vi "Get Logger Status.vi"(8 "Error In":errorcluster, 9 "Timeout (s)":dbl=10.0 format="%#_13g", 10 "Synchronize with Logger (False)":bool, 11 "TDMS Log In":refnum<class "TDMS Logger.lvclass">) -> (0 "Error Out":errorcluster, 1 "timed out?":bool, 2 "Logger Status":T1, 3 "TDMS Log Out":refnum<class "TDMS Logger.lvclass">)   [LabVIEW 2015, in "TDMS Logger.lvlib" / "TDMS Logger.lvclass"]
doc: "This VI returns the cluster with the status of the data logger. The status contains: number of files with the base name of this data logger, current log file size, current log file path, the start time of the current log file and the throughput of saving the current file.\n\nThe Synchronize with Logger input can be specified to true if the logger should first log all of the previous data before providing the status. If you set this input to TRUE you should provide large enough timeout for all the logging operations to complete.\n\nThe default value of the timeout is -1 which means that this VI will wait forever however if the Synchronize with Logger input is FALSE, the command to give status has high priority so in most situation the status will return quickly. The status will return slowly only when the previous packet that was to be logged was big and took a long time to log."
uses:
  TDMS Logger.lvclass
  _Typedefs/Logger Status Information.ctl
  TDMS Logger.lvclass/TDMS Logger.ctl
  _Typedefs/Log Message.ctl
  _Typedefs/Log Action.ctl
  _Typedefs/Data Type.ctl
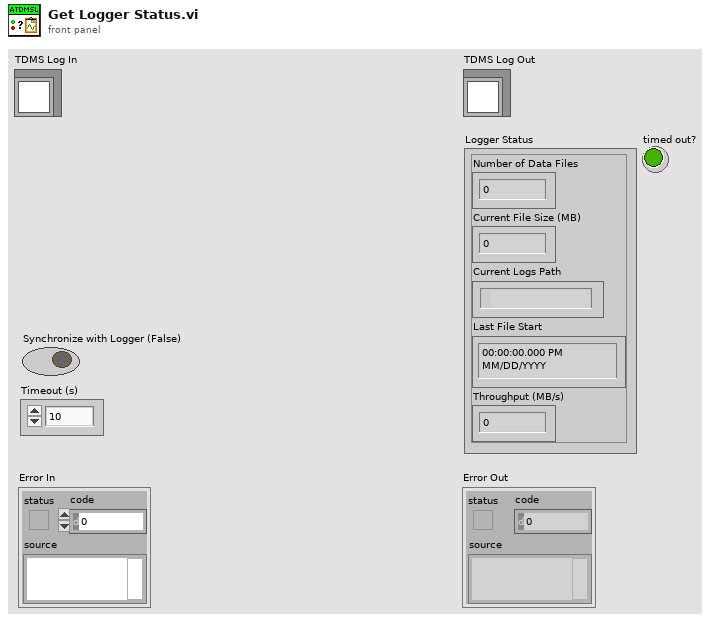
[diagram p1: front panel]
types:
  T1 = typedef "TDMS Logger.lvlib/TDMS Logger.lvclass/Logger Status Information.ctl" = cluster{"Number of Data Files":i32, "Current File Size (MB)":dbl, "Current Logs Path":path, "Last File Start":timestamp, "Throughput (MB/s)":dbl}
  T2 = typedef "TDMS Logger.lvlib/TDMS Logger.lvclass/Log Action.ctl" = enum16{"Handle Old Files", "Status Update", "Stop", "Log Data", "Initialize"}
  T3 = typedef "TDMS Logger.lvlib/TDMS Logger.lvclass/Log Message.ctl" = cluster{"Log Action":T2, "Variant":variant, "Data Type":T4, "Group Name":string, "Channels Names":string[]}
  T4 = typedef "TDMS Logger.lvlib/TDMS Logger.lvclass/Data Type.ctl" = enum16{"I16", "I8", "String", "U16", "U8", "Waveform", "Double", "Single"}
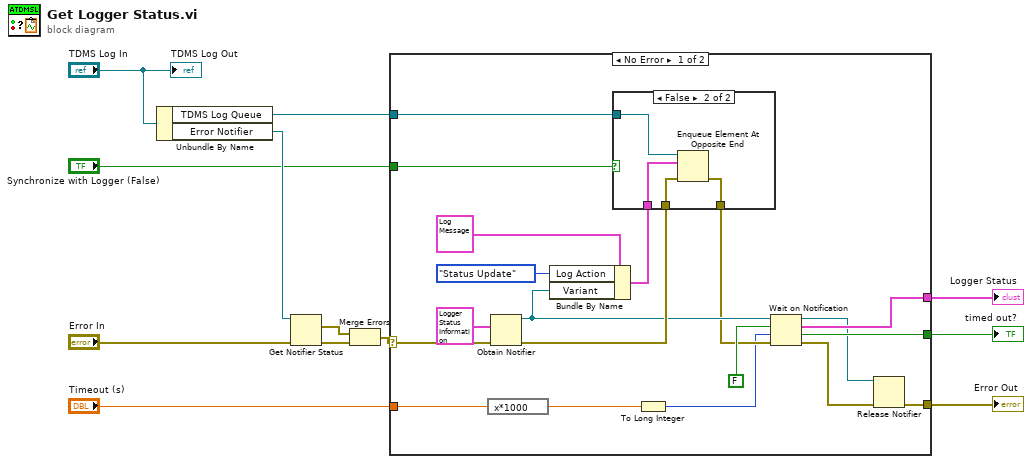
[diagram p0: block diagram]
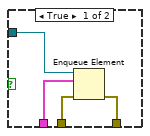
[diagram p2: hidden frame]
diagram:
  n1 = Unbundle By Name("TDMS Log In") -> ("TDMS Log Queue"=w11:refnum<queue>, "Error Notifier"=w9:refnum<notifier>)
  n2 = Get Notifier Status(notifier=w9, error in (no error)="Error In") -> (current notification=w7:errorcluster, error out=w8:errorcluster)  [unwired: 3 out]
  n3 = Merge Errors(w7, w8) -> (w1:errorcluster)
  n4 = case shown="No Error" w1 {
    selector: w1 -> [w27 w40]
    tunnel: [w20 w40] -> w12
    tunnel: w11 -> [w28 _]
    tunnel: "Timeout (s)" -> [w15 _]
    tunnel: [w23 _] -> w5
    tunnel: [w22 _] -> w4
    tunnel: "Synchronize with Logger (False)" -> [w16 _]
    frame No Error {
      n5 = expression code="x*1000"(w15) -> (w14:dbl)
      n6 = Obtain Notifier(notification data type=T1 {"Number of Data Files"=0, "Current File Size (MB)"=0.0, "Current Logs Path"=path "", "Last File Start"=timestamp(0 s since 1904-01-01), "Throughput (MB/s)"=0.0} ("Logger Status"), error in (no error)=w27) -> (notifier out=w24:refnum<notifier>, error out=w25:errorcluster)  [unwired: 2 in, 1 out]
      n7 = Bundle By Name(cluster=T3 {"Log Action"=enum."Stop", "Variant"=variant, "Data Type"=enum."String", "Group Name"="", "Channels Names"=[]} ("element"), "Log Action"=Log_Action."Status Update", "Variant"=w24) -> (w29:T3)
      n8 = case shown="False" w16 {
        tunnel: w29 -> [w35 w39]
        tunnel: w28 -> [w34 w38]
        tunnel: w25 -> [w33 w37]
        tunnel: [w32 w36] -> w19
        frame True {
          n9 = Enqueue Element(queue=w34, element=w35, error in (no error)=w33) -> (error out=w32:errorcluster)  [unwired: 1 in, 2 out]
        }
        frame False {
          n10 = Enqueue Element At Opposite End(queue=w38, element=w39, error in (no error)=w37) -> (error out=w36:errorcluster)  [unwired: 1 in, 2 out]
        }
      }
      n11 = To Long Integer(number=w14) -> (32bit integer=w13:i32)
      n12 = Wait on Notification(notifier=w24, ignore previous (F)=FALSE, timeout in ms (-1)=w13, error in (no error)=w19) -> (notifier out=w18:refnum<notifier>, notification=w23:T1, timed out?=w22:bool, error out=w17:errorcluster)
      n13 = Release Notifier(notifier=w18, error in (no error)=w17) -> (error out=w20:errorcluster)  [unwired: 1 in, 2 out]
    }
    frame Error {
    }
  }
  "Error Out" <- w12
  "Logger Status" <- w5
  "timed out?" <- w4
  "TDMS Log Out" <- "TDMS Log In"
